vi "GetAllCalTables(LTC20)V0.56.vi"(2 "error in (no error)":errorcluster, 3 "LTC-20 IEEE":refnum<visa-resource-name>) -> (0 "error out":errorcluster, 1 "CalTables":string[](array[string])=["Diode2V ;2;-1.;LS Diode #10;  n/a;\n", "Diode2V ;2;-1.;CryoCal D3;  n/a;\n", "Diode2V ;2;-1.;SI-410NN;  n/a;\n", "Diode6V ;2;1.;LS TG-120;  n/a;\n", "R250  DC;1;1.;PT100/385   ;  n/a;\n", "R2500 DC;1;10.;PT1000/385   ;  n/a;\n", "R250  DC;1;1.;PT100/392   ;  n/a;\n", "R2500 DC;1;10.;PT1000/392   ;  n/a;\n", "R1.0M AC;0;1.;Cal Res. 10mV; 10mV;\n", "R1.0M AC;0;1.;Cal Res. 3mV;  3mV;\n", "R1.0M AC;0;1.;Cal Res. 1mV ;  1mV;\n", "R1.0M AC;0;1.;Cal Res. 320uV;320uV;\n", "R1.0M AC;0;1.;Cal Res. 100uV;100uV;\n", "R1.0M AC;0;1.;Cal Res. 32uV; 32uV;\n", "R1.0M AC;0;1.;Cal Res. 10uV; 10uV;\n", "R1.0M AC;0;1.;cernoxX02509;  1mV;\n", "R1.0M AC;0;1.;#NMLCnx1050X01779;  1mV;\n", "R1.0M AC;0;1.;NMLCNX2512extrap;  1mV;\n", "R1.0M AC;0;1.;VSMcernoxx03872;  1mV;\n", "R1.0M AC;0;1.;OcernoxX02363; 10mV;\n", "R1.0M AC;0;1.;OcernoxX02158; 10mV;\n", "R1.0M AC;0;1.;#cw1050X03473;  3mV;\n", "R1.0M AC;0;1.;NMRX01906;  1mV;\n", "R1.0M AC;0;-1.;OptCernoxX02158;  1mV;\n", "R1.0M AC;0;-1.;OptCernoxX04981;  1mV;\n", "R1.0M AC;0;-1.;OptCernoxX02158;  1mV;\n"])   [LabVIEW 2019]
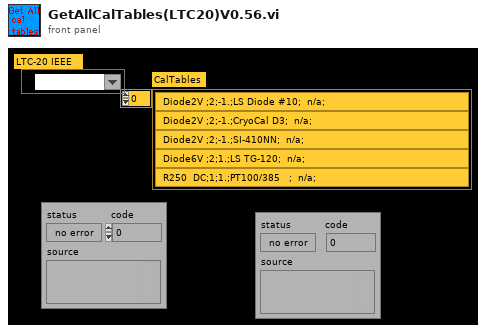
[diagram p1: front panel]
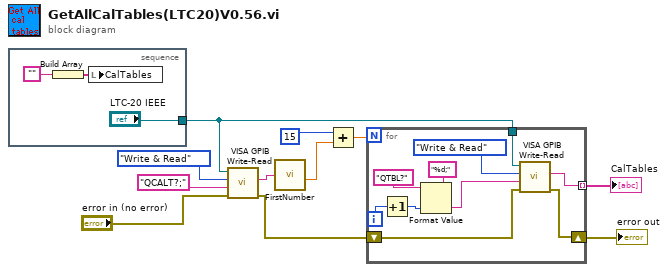
[diagram p0: block diagram]
diagram:
  n1 = stacked-sequence {
    tunnel: ["LTC-20 IEEE"] -> w1
    frame #0 {
      n2 = Build Array("") -> (w14:string[])
      n3 = local write "CalTables"(w14) -> ()
    }
  }
  n4 = call "VISA GPIB Write-Read.vi"("error in (no error)"="error in (no error)", "Command"="QCALT?;", "Action"=enum16{"Write", "Read", "Write & Read"}."Write & Read", "VISA resource name"=w1) -> ("error out"=w3:errorcluster, "String Returned"=w9:string)  [unwired: 4 in, 2 out]
  n5 = call "FirstNumber.vi"("Input String"=w9) -> ("FirstNumber"=w6:ext)  [unwired: 5 out]
  n6 = Add(x=15, y=w6) -> (x+y=w5:ext)
  n7 = for {
    N: w5 -> [_]
    tunnel: [w19] -> w11 mode=indexing
    tunnel: w1 -> [w15]
    shift-right: [w16] -> w2
    shift-left: w3 -> [w17]
    i -> [w24]
    n8 = Increment(x=w24) -> (x+1=w23:i32)
    n9 = Format Value(string ("")="QTBL?", format string="%d;", value (0)=w23) -> (output string=w20:string)
    n10 = call "VISA GPIB Write-Read.vi"("error in (no error)"=w17, "Command"=w20, "Action"=enum16{"Write", "Read", "Write & Read"}."Write & Read", "VISA resource name"=w15) -> ("error out"=w16:errorcluster, "String Returned"=w19:string)  [unwired: 4 in, 2 out]
  }
  "CalTables" <- w11
  "error out" <- w2
